vi "Server_Connection Manager(FGV).vi"(6 "Connection Manager Method(Get)":T3=enum."Get", 8 "error in":errorcluster, 10 "Connection Properties In":T1={"User Data"={"Name"="", "Email"="", "Phone Number"="", "User Picture"=array225x225[50625 elements], "Last Login Time"=timestamp(0 s since 1904-01-01)}, "Data"={"t0"=timestamp(0 s since 1904-01-01), "dt"=1.0, "Y"=[]}}, 11 "Connection In":refnum<k5>) -> (0 "error out":errorcluster, 1 "All Connections":refnum<k5>[](array[refnum]), 2 "Connection Properties Out":T1={"User Data"={"Name"="", "Email"="", "Phone Number"="", "User Picture"=array225x225[50625 elements], "Last Login Time"=timestamp(0 s since 1904-01-01)}, "Data"={"t0"=timestamp(0 s since 1904-01-01), "dt"=1.0, "Y"=[]}}, 3 "Connection Out":refnum<k5>, 5 "All Connection Properties":T1[](array[typedef]))   [LabVIEW 2018, in "Cloud Server.lvlib"]
doc: "宣告客端連線ID和使用者資訊的佔存記憶體"
uses:
  Cloud Server.lvlib
  Data Def/Server_Connection Manager Method.ctl
  Data Def/Server_Connection Properties.ctl
  Com VIs/Data Def/User Data.ctl
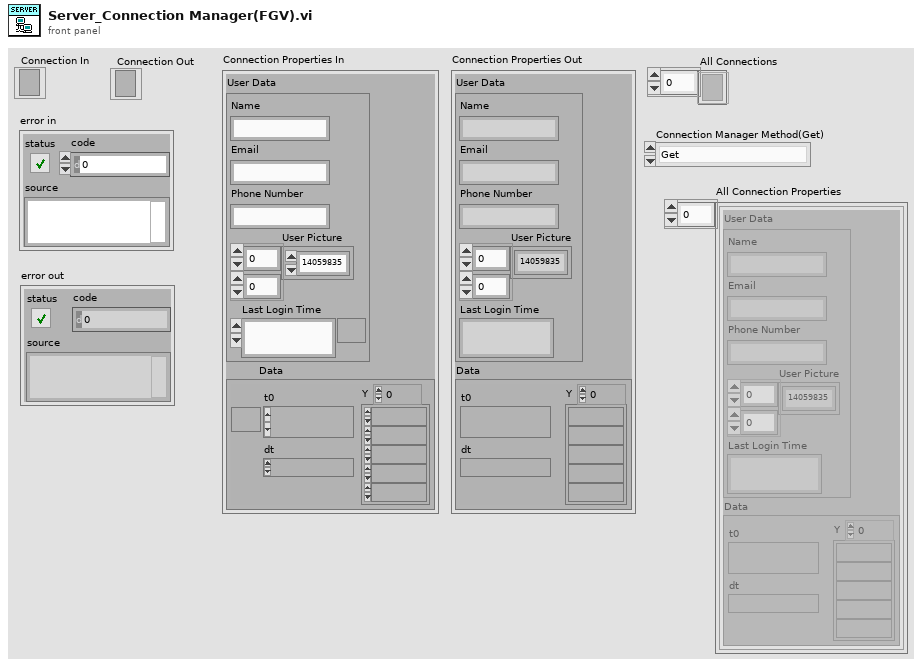
[diagram p1: front panel]
types:
  T1 = typedef "Cloud Server.lvlib/Server_Connection Properties.ctl" = cluster{"User Data":T2, "Data":waveform(dbl)}
  T2 = typedef "User Data.ctl" = cluster{"Name":string, "Email":string, "Phone Number":string, "User Picture":u32[][], "Last Login Time":timestamp}
  T3 = typedef "Cloud Server.lvlib/Server_Connection Manager Method.ctl" = enum16{"Initialize", "Add", "Get", "Set Properties", "Get Properties", "Close", "Release"}
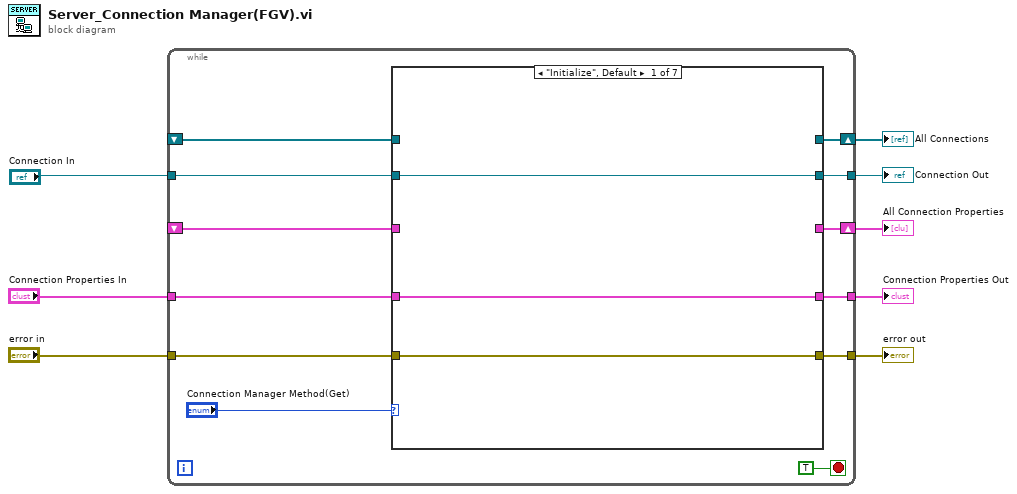
[diagram p0: block diagram]
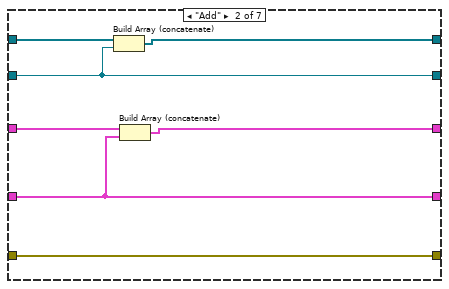
[diagram p2: hidden frame]
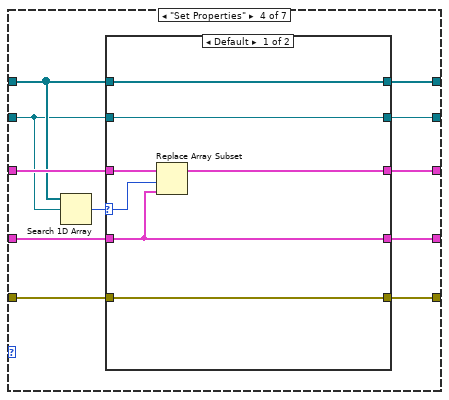
[diagram p4: hidden frame]
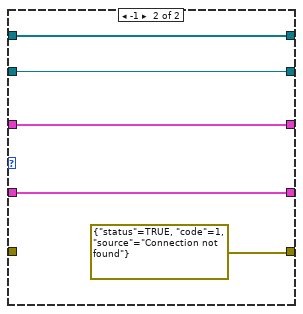
[diagram p5: hidden frame]
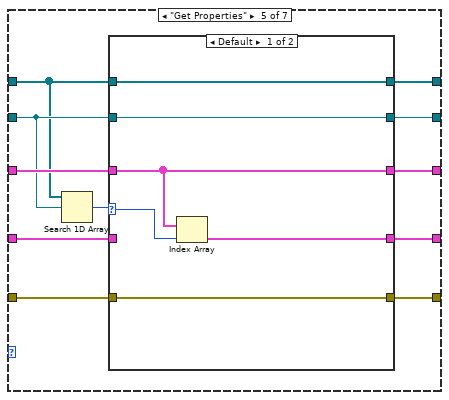
[diagram p6: hidden frame]
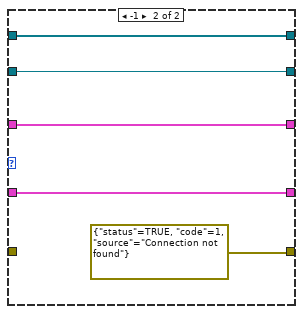
[diagram p7: hidden frame]
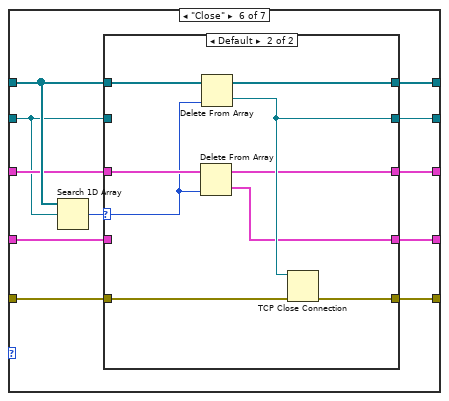
[diagram p8: hidden frame]
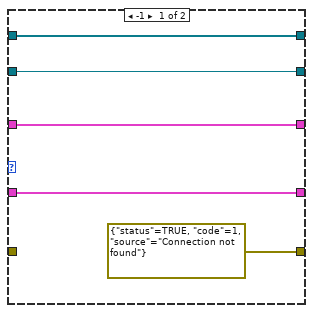
[diagram p9: hidden frame]
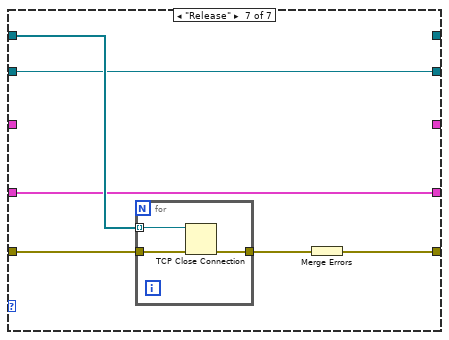
[diagram p10: hidden frame]
diagram:
  n1 = while {
    tunnel: "Connection In" -> [w18]
    tunnel: [w17] -> w5
    shift-right: [w16] -> w3
    shift-left: _ -> [w15]
    tunnel: "Connection Properties In" -> [w14]
    shift-right: [w13] -> w4
    shift-left: _ -> [w12]
    tunnel: [w11] -> w6
    tunnel: "error in" -> [w10]
    tunnel: [w9] -> w1
    stop <- TRUE stop-if-true
    n2 = case shown="\"Initialize\", Default" "Connection Manager Method(Get)" {
      tunnel: w18 -> [w23 w30 w34 w37 w66 w83 w107]
      tunnel: [w23 w30 w34 w36 w63 w88 w107] -> w17
      tunnel: [_ w29 w35 w38 w64 w91 _] -> w16
      tunnel: w15 -> [_ w28 w35 w39 w65 w90 w108]
      tunnel: w14 -> [w22 w25 w32 w42 w68 w82 w106]
      tunnel: [_ w27 w33 w41 w62 w85 _] -> w13
      tunnel: w12 -> [_ w26 w33 w43 w67 w87 _]
      tunnel: [w22 w25 w32 w40 w61 w81 w106] -> w11
      tunnel: w10 -> [w21 w24 w31 w45 w69 w84 w111]
      tunnel: [w21 w24 w31 w44 w60 w86 w109] -> w9
      frame "Initialize", Default {
      }
      frame "Add" {
        n3 = Build Array (concatenate)(w28, w30) -> (w29:refnum<k5>[])
        n4 = Build Array (concatenate)(w26, w25) -> (w27:T1[])
      }
      frame "Get" {
      }
      frame "Set Properties" {
        n5 = Search 1D Array(1D array=w39, element=w37) -> (index of element=w46:i32)  [unwired: 1 in]
        n6 = case shown="Default" w46 {
          selector: w46 -> [w52 _]
          tunnel: w45 -> [w47 _]
          tunnel: [w47 errorcluster {"status"=TRUE, "code"=1, "source"="Connection not found"} ("error out 2")] -> w44
          tunnel: w43 -> [w53 w58]
          tunnel: w42 -> [w50 w57]
          tunnel: [w51 w58] -> w41
          tunnel: [w50 w57] -> w40
          tunnel: w39 -> [w49 w56]
          tunnel: [w49 w56] -> w38
          tunnel: w37 -> [w48 w55]
          tunnel: [w48 w55] -> w36
          frame Default {
            n7 = Replace Array Subset(array=w53, new element=w50, index=w52) -> (w51:T1[])
          }
          frame -1 {
          }
        }
      }
      frame "Get Properties" {
        n8 = Search 1D Array(1D array=w65, element=w66) -> (index of element=w59:i32)  [unwired: 1 in]
        n9 = case shown="Default" w59 {
          selector: w59 -> [w72 _]
          tunnel: w69 -> [w73 _]
          tunnel: [w73 errorcluster {"status"=TRUE, "code"=1, "source"="Connection not found"} ("error out 2")] -> w60
          tunnel: w67 -> [w71 w80]
          tunnel: w68 -> [_ w79]
          tunnel: [w71 w80] -> w62
          tunnel: [w70 w79] -> w61
          tunnel: w65 -> [w75 w78]
          tunnel: [w75 w78] -> w64
          tunnel: w66 -> [w74 w77]
          tunnel: [w74 w77] -> w63
          frame Default {
            n10 = Index Array(array=w71, index=w72) -> (element=w70:T1)
          }
          frame -1 {
          }
        }
      }
      frame "Close" {
        n11 = Search 1D Array(1D array=w90, element=w83) -> (index of element=w89:i32)  [unwired: 1 out]
        n12 = case shown="Default" w89 {
          selector: w89 -> [_ w99]
          tunnel: w90 -> [w96 w104]
          tunnel: [w96 w105] -> w91
          tunnel: [w94 w103] -> w88
          tunnel: w87 -> [w95 w101]
          tunnel: [errorcluster {"status"=TRUE, "code"=1, "source"="Connection not found"} ("error out 2") w102] -> w86
          tunnel: [w95 w100] -> w85
          tunnel: w84 -> [_ w98]
          tunnel: w83 -> [w94 _]
          tunnel: w82 -> [w92 _]
          tunnel: [w92 w97] -> w81
          frame -1 {
          }
          frame Default {
            n13 = Delete From Array(array=w101, index=w99) -> (deleted portion=w97:T1, array with subset deleted=w100:T1[])  [unwired: 1 in]
            n14 = Delete From Array(array=w104, index=w99) -> (deleted portion=w103:refnum<k5>, array with subset deleted=w105:refnum<k5>[])  [unwired: 1 in]
            n15 = TCP Close Connection(connection ID=w103, error in (no error)=w98) -> (error out=w102:errorcluster)  [unwired: 2 out]
          }
        }
      }
      frame "Release" {
        n16 = for {
          tunnel: w111 -> [w114]
          tunnel: [w113] -> w110
          tunnel: w108 -> [w112] mode=indexing
          n17 = TCP Close Connection(connection ID=w112, error in (no error)=w114) -> (error out=w113:errorcluster)  [unwired: 1 in, 1 out]
        }
        n18 = Merge Errors(w110) -> (w109:errorcluster)
      }
    }
  }
  "Connection Out" <- w5
  "error out" <- w1
  "All Connections" <- w3
  "All Connection Properties" <- w4
  "Connection Properties Out" <- w6
